vi "Vision Research Phantom Series PhCon PhGetCineStatus.vi"(0 "CN in":u32, 5 "Error In (no error)":errorcluster, 8 "Simulate? (False)":bool) -> (14 "CN out":u32=1, 16 "pCS":T1[](array[typedef]), 19 "Error Out":errorcluster)   [LabVIEW 2013, in "VRI.lvlib"]
doc: "PhCon.dll\n\nPhGetCineStatus\nHRESULT PhGetCineStatus(UINT CN, PCINESTATUS pCS);\n\nParameters Description\nCN (in) Camera number.\npCineStatus(out) Array of CINESTATUS structures for all the defined cines \n containing information whether the recording is finished, \n the trigger was received or the Cine is just recording now. \n This buffer have to be allocated for MAXCINECNT cines.\nReturn HRESULT (0=Ok)\nComments Check the status of all the cines defined in the camera \n (finished, active, triggered)."
uses:
  VRI.lvlib
  _Type Defs/PHCon CINESTATUS.ctl
  Phantom DLLs/PhCon.dll
panel:
  # "For instructions on the use of this VI, press Ctrl+H to display the help window and move the mouse over the icon, controls, and indicators"
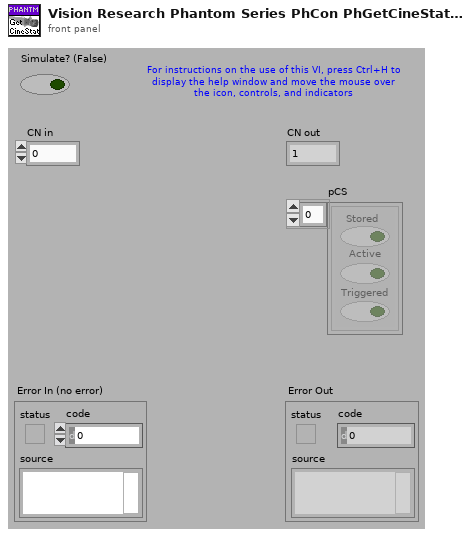
[diagram p1: front panel]
types:
  T1 = typedef "VRI.lvlib/PHCon CINESTATUS.ctl" = cluster{"Stored":bool, "Active":bool, "Triggered":bool}
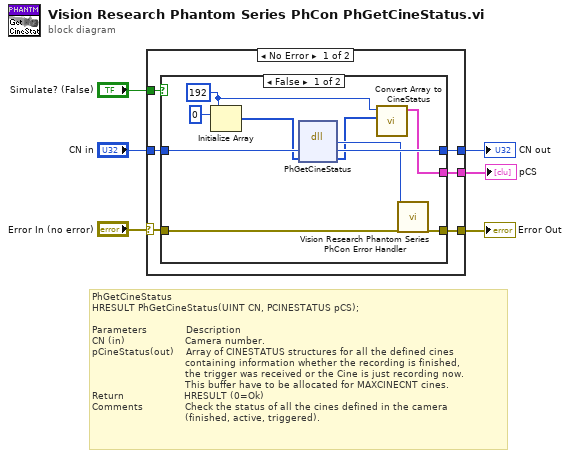
[diagram p0: block diagram]
diagram:
  # "PhGetCineStatus\nHRESULT PhGetCineStatus(UINT CN, PCINESTATUS pCS);\n\nParameters             Description\nCN (in)                    Camera number.\npCineStatus(out)    Array of CINESTATUS structures for all the defined cines                                                                              \n                               containing information whether the recording is finished, \n                               the trigger was received or the Cine is just recording now. \n                               This buffer have to be allocated for MAXCINECNT cines.\nReturn                    HRESULT (0=Ok)\nComments              Check the status of all the cines defined in the camera \n                               (finished, active, triggered)."
  n1 = case shown="No Error" "Error In (no error)" {
    selector: "Error In (no error)" -> [w12 w26]
    tunnel: [w11 w26] -> w5
    tunnel: "Simulate? (False)" -> [w10 _]
    tunnel: "CN in" -> [w9 w25]
    tunnel: [w8 w25] -> w2
    tunnel: [w7 _] -> w1
    frame No Error {
      n2 = case shown="False" w10 {
        tunnel: w12 -> [w21 w24]
        tunnel: [w22 w24] -> w11
        tunnel: w9 -> [w20 w23]
        tunnel: [w19 w23] -> w8
        tunnel: [w13 _] -> w7
        frame False {
          w14 = u32 192 ("dimension size")
          n3 = Initialize Array(u32 0 ("element"), w14) -> (w16:u32[])
          n4 = dll-call lib="C:/Projects/SDK/32-bit/Vision Research Phantom Series Labview Driver/Phantom DLLs/PhCon.dll" fn="PhGetCineStatus"("CN"=w20, "pCS"=w16) -> ("HRESULT"=w18:i32, "CN"=w19:u32, "pCS"=w15:u32[])  [unwired: 3 in, 2 out]
          n5 = call "Convert Array to CineStatus.vi"("pCS array"=w15, "Numeric"=w14) -> ("pCS out"=w13:T1[])  [unwired: 9 out]
          n6 = call "Vision Research Phantom Series PhCon Error Handler.vi"("ErrNo"=w18, "Error In (no error)"=w21) -> ("Error Out"=w22:errorcluster)  [unwired: 17 out]
        }
        frame True {
          # "It looks as though the dlls can provide simulated data so this case may not have to be used"
        }
      }
    }
    frame Error {
    }
  }
  "Error Out" <- w5
  "CN out" <- w2
  "pCS" <- w1
